vi "Get Rx IPs and Ports.vi"(0 "Target Names":string[](array[string])=["AE-HIL-1", "AE-HIL-2", "AE-HIL-3"], 1 "IP Addresses":string[](array[string])=["169.254.239.43", "169.254.184.119", "169.254.184.0"], 7 "Remote Target Name":string="AE-HIL-2", 13 "Local Target Index":i32) -> (4 "Local IP Address":string="169.254.239.43", 6 "Local Port Number":string="1000", 10 "Remote IP Address":string, 15 "Remote Port Number":string="1000")   [LabVIEW 2023]
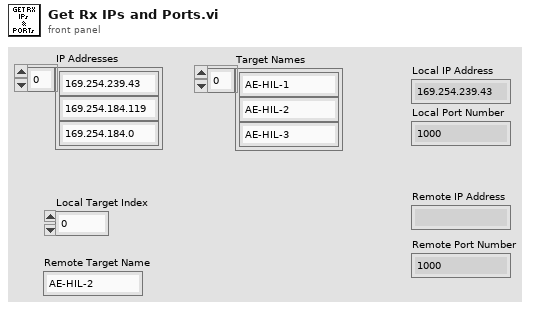
[diagram p1: front panel]
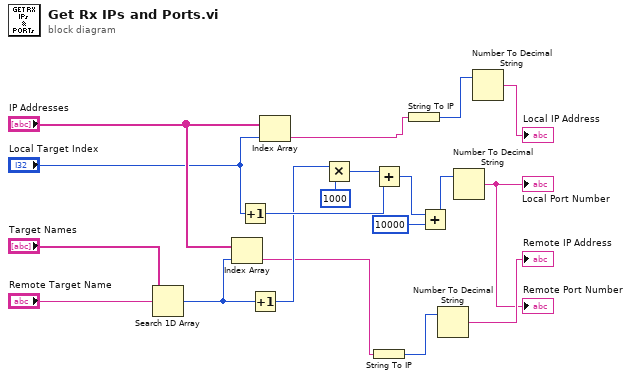
[diagram p0: block diagram]
diagram:
  n1 = Search 1D Array(1D array="Target Names", element="Remote Target Name") -> (index of element=w14:i32)  [unwired: 1 in]
  n2 = Index Array(array="IP Addresses", index=w14) -> (element=w5:string)
  n3 = Increment(x="Local Target Index") -> (x+1=w12:i32)
  n4 = Increment(x=w14) -> (x+1=w11:i32)
  n5 = Index Array(array="IP Addresses", index="Local Target Index") -> (element=w8:string)
  n6 = Multiply(x=w11, y=1000) -> (x*y=w16:i32)
  n7 = Add(x=w16, y=w12) -> (x+y=w3:i32)
  n8 = String To IP(1:w5) -> (0:w6:u32)
  n9 = String To IP(1:w8) -> (0:w9:u32)
  n10 = Add(x=w3, y=10000) -> (x+y=w1:i32)
  n11 = Number To Decimal String(number=w6) -> (decimal integer string=→"Remote IP Address":string)  [unwired: 1 in]
  n12 = Number To Decimal String(number=w1) -> (decimal integer string=→"Local Port Number" →"Remote Port Number":string)  [unwired: 1 in]
  n13 = Number To Decimal String(number=w9) -> (decimal integer string=→"Local IP Address":string)  [unwired: 1 in]
